vi "To DateTime Array.vi"(1 "Formatted DateTime Array":dbl[](array[numeric])) -> (0 "DateTime Array":timestamp[](array[timestamp]))   [LabVIEW 2013, in "OPC UA runtime.lvclass"]
doc: "Convert array of DCAF tags to DateTime format which can be used by OPC UA functions."
uses:
  OPC UA runtime.lvclass
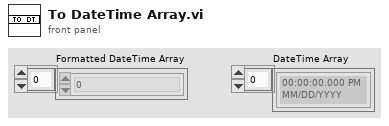
[diagram p1: front panel]
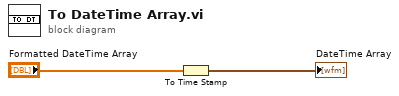
[diagram p0: block diagram]
diagram:
  n1 = To Time Stamp(1:"Formatted DateTime Array") -> (0:→"DateTime Array":timestamp[])
